vi "Process var.vi"() -> ()   [LabVIEW 2016]
panel:
  out "CODcr参数输出":T1 {"跨度参数输出"."mean" format="%0.2f"; "零点参数输出"."mean" format="%0.2f"; "水样参数输出"."mean" format="%0.2f"}
  out "CODMn参数输出":T1 {"跨度参数输出"."mean" format="%0.2f"; "零点参数输出"."mean" format="%0.2f"; "水样参数输出"."mean" format="%0.2f"}
  out "TN参数输出":T1 {"跨度参数输出"."mean" format="%0.2f"; "零点参数输出"."mean" format="%0.2f"; "水样参数输出"."mean" format="%0.2f"}
  out "TP参数输出":T1 {"跨度参数输出"."mean" format="%0.2f"; "零点参数输出"."mean" format="%0.2f"; "水样参数输出"."mean" format="%0.2f"}
  out "NH3N参数输出":T1 {"跨度参数输出"."mean" format="%0.2f"; "零点参数输出"."mean" format="%0.2f"; "水样参数输出"."mean" format="%0.2f"}
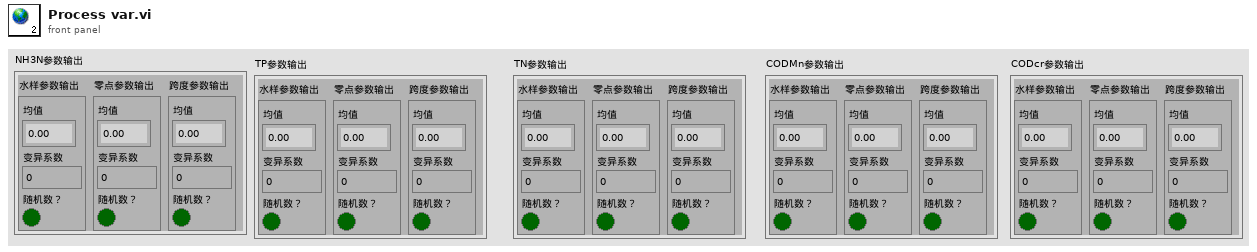
[diagram p1: front panel]
types:
  T1 = cluster{"水样参数输出":cluster{"mean":dbl, "变异系数":dbl, "随机数？":bool}, "零点参数输出":cluster{"mean":dbl, "变异系数":dbl, "随机数？":bool}, "跨度参数输出":cluster{"mean":dbl, "变异系数":dbl, "随机数？":bool}}
diagram:
